vi "Play_avi.vi"() -> ()   [LabVIEW 2019]
uses:
  <vilib>/vision/NI_Vision_Development_Module.lvlib
panel:
  in  "Replace Value":sgl=1.0 format="%.2f"
  out "Waveform Chart":cluster{u64, u64}(graph)
  out "Right lane":u8[][](graph)
  out "Left lane":u8[][](graph)
  out "ROI":T1={"Global Rectangle"=[72, 229, 702, 293], "Contours"=[{"Contour Type"=0, "ROI Type"=3, "Points"=[72, 229, 702, 293]}]}
  in  "Range":cluster{"Lower value":sgl, "Upper value":sgl}={"Lower value"=124.0, "Upper value"=255.0} {"Upper value" format="%.2f"; "Lower value" format="%.2f"}
  out "Image_binary":T2(plugin-control)
  out "Image_gray":T2(plugin-control)
  in  "Clamp Settings":T3={"Contrast"=47, "Filter width"=21, "Steepness"=10, "Subsampling Ratio"=20, "Show Search Area"=TRUE, "Show Search Lines"=TRUE, "Show Edges Found"=TRUE, "Show Result"=TRUE}
  in  "AVI File Path":path=path "C:/AGV/Log/0812/pusan_track_0812-2.avi"
  out "Image_color":T2(plugin-control)
  in  "Stop":bool=TRUE
  out "Progress Bar":i32(slide)=1110 max=1762 scale=-1.0..1762.0
  # "0812-2, 72,255"
  # "122,255"
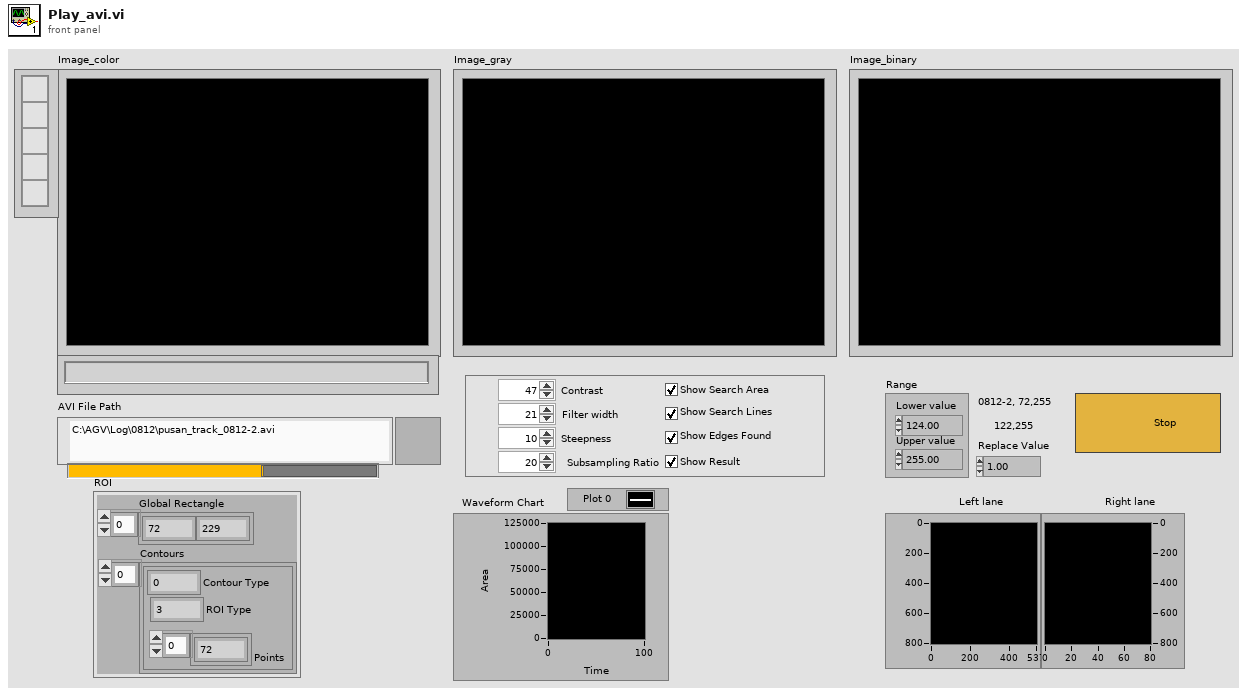
[diagram p1: front panel]
types:
  T1 = cluster{"Global Rectangle":i32[], "Contours":cluster{"Contour Type":u32, "ROI Type":u32, "Points":i32[]}[]}
  T2 = typedef "IMAQ Image.ctl" = refnum<image>
  T3 = cluster{"Contrast":i32, "Filter width":i32, "Steepness":i32, "Subsampling Ratio":u32, "Show Search Area":bool, "Show Search Lines":bool, "Show Edges Found":bool, "Show Result":bool}
  T4 = typedef "IMAQ AVI2 Refnum.ctl" = refnum<k20>
  T5 = typedef "Image Type" = u32
  T6 = cluster{"Width":u32, "Height":u32, "Frames Per Second":u32, "Codec":string, "Has Data":bool}
  T7 = cluster{"Clamp Settings":cluster{"Contrast":i32, "Filter width":i32, "Steepness":i32, "Subsampling Ratio":u32, "Show Search Area":bool, "Show Search Lines":bool, "Show Edges Found":bool, "Show Result":bool}, "Threshold":cluster{dbl, dbl}}
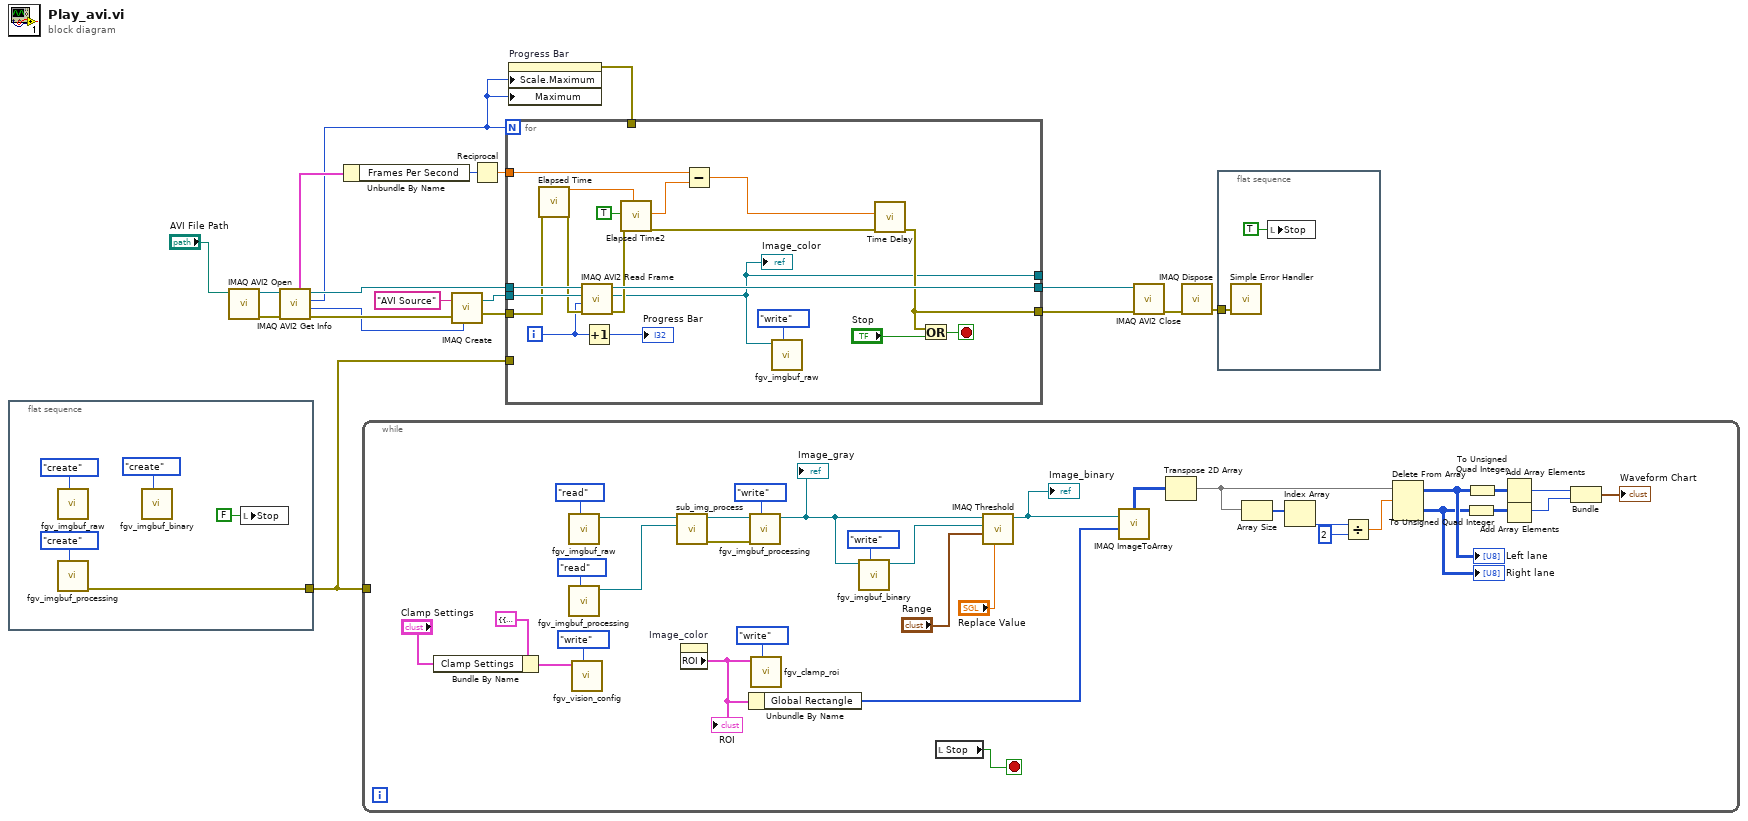
[diagram p0: block diagram]
diagram:
  n1 = flat-sequence {
    tunnel: [w22] -> w1
    frame #0 {
      n2 = call "fgv_imgbuf_raw.vi"("cmd"=enum16{"create", "close", "write", "read"}."create") -> ()  [unwired: 9 in, 2 out]
      n3 = call "fgv_imgbuf_processing.vi"("cmd"=enum16{"create", "close", "write", "read"}."create") -> ("error out"=w22:errorcluster)  [unwired: 9 in, 1 out]
      n4 = call "fgv_imgbuf_binary.vi"("cmd"=enum16{"create", "close", "write", "read"}."create") -> ()  [unwired: 9 in, 2 out]
      n5 = local write "Stop"(FALSE ("Stop")) -> ()
    }
  }
  n6 = call "IMAQ AVI2 Open"("AVI File Path"="AVI File Path") -> ("error out"=w16:errorcluster, "AVI Refnum"=w15:T4)  [unwired: 2 in, 7 out]
  n7 = call "IMAQ AVI2 Get Info"("error in (no error)"=w16, "AVI Refnum"=w15) -> ("error out"=w12:errorcluster, "Image Type"=w7:T5, "Number of Frames"=w4:u32, "AVI Refnum (duplicate)"=w9:T4, "Frame Data"=w17:T6)  [unwired: 5 out]
  n8 = Unbundle By Name(w17) -> ("Frames Per Second"=w6:u32)
  n9 = while {
    tunnel: w1 -> [_]
    stop <- w52 stop-if-true
    n10 = Bundle By Name(cluster=T7 {"Clamp Settings"={"Contrast"=44, "Filter width"=8, "Steepness"=8, "Subsampling Ratio"=12, "Show Search Area"=TRUE, "Show Search Lines"=TRUE, "Show Edges Found"=TRUE, "Show Result"=TRUE}, "Threshold"={0.0, 6.053639846743295}} ("Vison cfg out"), "Clamp Settings"="Clamp Settings") -> (w39:T7)
    n11 = call "fgv_imgbuf_raw.vi"("cmd"=enum16{"create", "close", "write", "read"}."read") -> ("Image"=w56:T2)  [unwired: 9 in, 1 out]
    n12 = call "fgv_imgbuf_processing.vi"("cmd"=enum16{"create", "close", "write", "read"}."read") -> ("Image"=w55:T2)  [unwired: 9 in, 1 out]
    n13 = call "fgv_vision_config.vi"("cmd"=enum16{"init", "read", "write"}."write", "Vison cfg"=w39) -> ()  [unwired: 8 in, 2 out]
    n14 = call "sub_img_process.vi"("Green or Sat Plane"=w55, "Image Src"=w56) -> ("error out"=w49:errorcluster, "Image Dst Out"=w53:T2)  [unwired: 8 in]
    n15 = property on="Image_color" class="ImageControl"() -> ("ROI"=w43:T1)  [unwired: 2 in, 2 out]
    "ROI" <- w43
    n16 = Unbundle By Name(w43) -> ("Global Rectangle"=w42:i32[])
    n17 = call "fgv_imgbuf_processing.vi"("cmd"=enum16{"create", "close", "write", "read"}."write", "error in"=w49, "raw Image in"=w53) -> ("Image"=w46:T2)  [unwired: 7 in, 1 out]
    "Image_gray" <- w46
    n18 = call "fgv_clamp_roi.vi"("cmd"=enum16{"init", "read", "write"}."write", "ROI-clamp"=w43) -> ()  [unwired: 9 in, 1 out]
    n19 = call "fgv_imgbuf_binary.vi"("cmd"=enum16{"create", "close", "write", "read"}."write", "raw Image in"=w46) -> ("raw image out"=w47:T2)  [unwired: 8 in, 1 out]
    n20 = local read "Stop"() -> (w52:bool)
    n21 = call "IMAQ Threshold"("Replace Value"="Replace Value", "Range"="Range", "Image Dst"=w47, "Image Src"=w46) -> ("Image Dst Out"=w44:T2)  [unwired: 6 in, 1 out]
    "Image_binary" <- w44
    n22 = call "IMAQ ImageToArray"("Optional Rectangle"=w42, "Image"=w44) -> ("Image Pixels (U8)"=w38:u8[][])  [unwired: 2 in, 4 out]
    n23 = Transpose 2D Array(2D array=w38) -> (transposed array=w26:u8[][])
    n24 = Array Size(array=w26) -> (size(s)=w37:i32[])
    n25 = Index Array(array=w37) -> (element=w36:i32)  [unwired: 1 in]
    n26 = Divide(x=w36, y=2) -> (x/y=w34:dbl)
    n27 = Delete From Array(array=w26, length=w34) -> (deleted portion=w32:u8[][], array with subset deleted=w33:u8[][])  [unwired: 2 in]
    "Left lane" <- w33
    "Right lane" <- w32
    n28 = To Unsigned Quad Integer(1:w32) -> (0:w28:u64[][])
    n29 = To Unsigned Quad Integer(1:w33) -> (0:w27:u64[][])
    n30 = Add Array Elements(numeric array=w27) -> (sum=w29:u64)
    n31 = Add Array Elements(numeric array=w28) -> (sum=w30:u64)
    n32 = Bundle(w29, w30) -> (→"Waveform Chart":cluster{u64, u64})  [unwired: 1 in]
  }
  n33 = call "IMAQ Create"("Image Name"="AVI Source", "Image Type"=w7, "error in (no error)"=w12) -> ("New Image"=w10:T2, "error out"=w11:errorcluster)  [unwired: 1 in, 1 out]
  n34 = Reciprocal(x=w6) -> (1/x=w5:dbl)
  n35 = property on="Progress Bar" class="Slide (엄격한)"("Scale.Maximum"=w4, "Maximum"=w4) -> (error out=w3:errorcluster)  [unwired: 2 in, 1 out]
  n36 = for {
    N: w4 -> [_]
    tunnel: w10 -> [w76]
    tunnel: [w75] -> w13
    tunnel: [w65] -> w14
    tunnel: w11 -> [w74]
    tunnel: w9 -> [w77]
    tunnel: [w59] -> _
    tunnel: w5 -> [w72]
    tunnel: w3 -> [_]
    tunnel: w1 -> [_]
    i -> [w62]
    stop <- w63 stop-if-true
    n37 = call "Elapsed Time"("error in (no error)"=w74) -> ("Present (s)"=w70:dbl, "error out"=w73:errorcluster)  [unwired: 11 in, 6 out]
    n38 = call "IMAQ AVI2 Read Frame"("error in (no error)"=w73, "Frame Number"=w62, "Image"=w76, "AVI Refnum"=w77) -> ("error out"=w68:errorcluster, "Image Out"=w59:T2, "AVI Refnum (duplicate)"=w75:T4)  [unwired: 5 out]
    "Image_color" <- w59
    n39 = Increment(x=w62) -> (x+1=→"Progress Bar":i32)
    n40 = call "Elapsed Time2"("Reset"=TRUE, "error in (no error)"=w68, "Set Start Time (s)"=w70) -> ("Elapsed Time (s)"=w67:dbl, "error out"=w66:errorcluster)  [unwired: 9 in, 6 out]
    n41 = Subtract(x=w72, y=w67) -> (x-y=w71:dbl)
    n42 = call "fgv_imgbuf_raw.vi"("cmd"=enum16{"create", "close", "write", "read"}."write", "raw Image in"=w59) -> ()  [unwired: 8 in, 2 out]
    n43 = call "Time Delay"("error in (no error)"=w66, "Delay Time (s)"=w71) -> ("error out"=w65:errorcluster)  [unwired: 9 in]
    n44 = Or(x=w65, y="Stop") -> (x .or. y?=w63:bool)
  }
  n45 = call "IMAQ AVI2 Close"("error in (no error)"=w14, "AVI Refnum"=w13) -> ("error out"=w8:errorcluster)  [unwired: 9 out]
  n46 = call "IMAQ Dispose"("error in (no error)"=w8) -> ("error out"=w18:errorcluster)  [unwired: 2 in, 3 out]
  n47 = flat-sequence {
    tunnel: w18 -> [w79]
    frame #0 {
      n48 = call <vilib>:"Simple Error Handler.vi"("error in (no error)"=w79) -> ()  [unwired: 1 in, 8 out]
      n49 = local write "Stop"(TRUE ("Stop")) -> ()
    }
  }
